vi "Find Controls Log Files for Shift.vi"(8 "error in (no error)":errorcluster, 10 "Date/Time":T1, 11 "Log File Directory":path=path "C:/Users/plane/Desktop/Data/runs-2014_11_21_16_00/runs") -> (0 "error out":errorcluster, 3 "Relevant Log Files":path[](array[path]))   [LabVIEW 2013, in "Controls Log Monitor.lvlib"]
uses:
  <vilib>/Utility/miscctls.llb/LVDateTimeRec.ctl
  Controls Log Monitor.lvlib
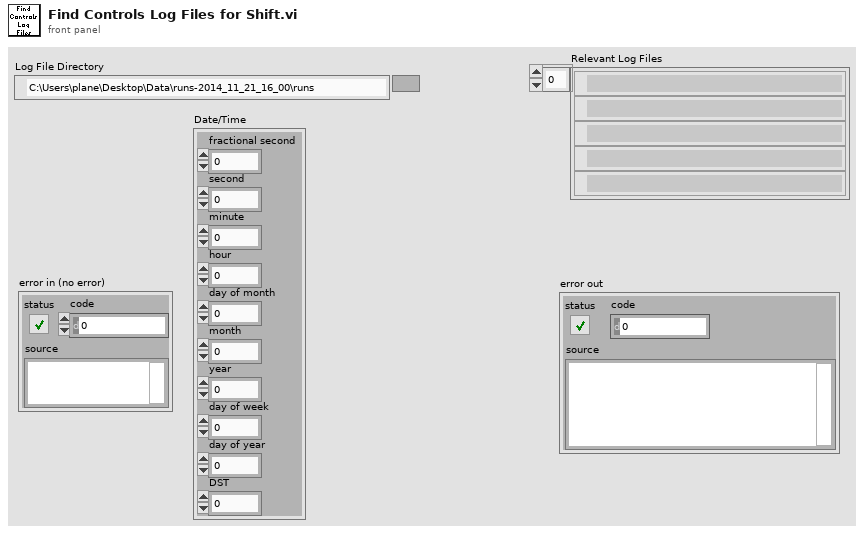
[diagram p1: front panel]
types:
  T1 = typedef "LVDateTimeRec.ctl" = cluster{"fractional second":dbl, "second":i32, "minute":i32, "hour":i32, "day of month":i32, "month":i32, "year":i32, "day of week":i32, "day of year":i32, "DST":i32}
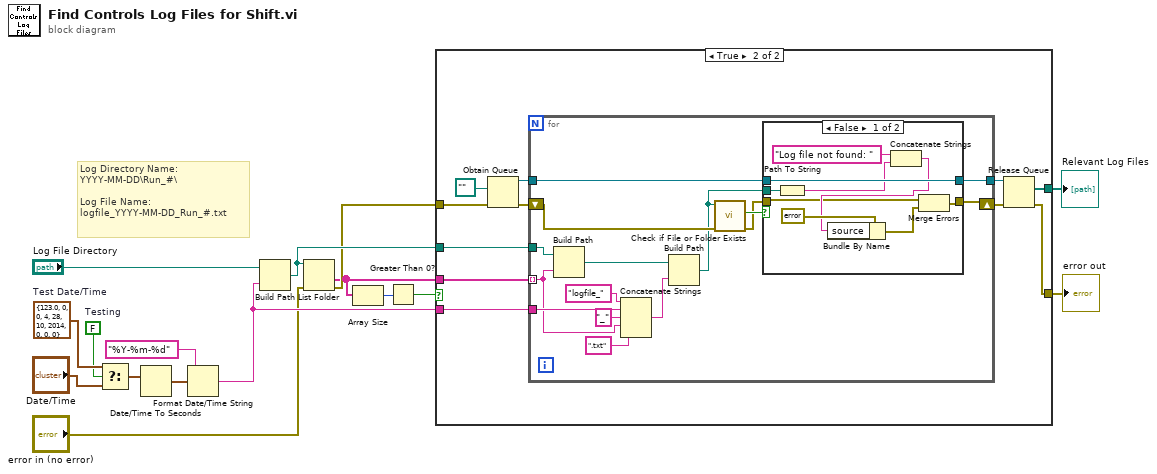
[diagram p0: block diagram]
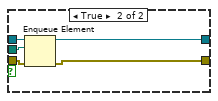
[diagram p3: hidden frame]
diagram:
  w7 = FALSE  # Testing
  w8 = T1 {"fractional second"=123.0, "second"=0, "minute"=0, "hour"=4, "day of month"=28, "month"=10, "year"=2014, "day of week"=0, "day of year"=0, "DST"=0}  # Test Date/Time
  # "Log Directory Name:\nYYYY-MM-DD\\Run_#\\\n\nLog File Name:\nlogfile_YYYY-MM-DD_Run_#.txt"
  n1 = Select(t=w8, s=w7, f="Date/Time") -> (s? t:f=w10:T1)
  n2 = Date/Time To Seconds(2:w10) -> (0:w16:timestamp)  [unwired: 1 in]
  n3 = Format Date/Time String(time format string (%c)="%Y-%m-%d", seconds (now)=w16) -> (date/time string=w12:string)  [unwired: 1 in]
  n4 = Build Path(base path="Log File Directory", name or relative path=w12) -> (appended path=w13:path)
  n5 = List Folder(path=w13, error in="error in (no error)") -> (folder names=w3:string[], error out=w5:errorcluster)  [unwired: 2 in, 2 out]
  n6 = Array Size(array=w3) -> (size(s)=w2:i32)
  n7 = Greater Than 0?(x=w2) -> (x > 0?=w1:bool)
  n8 = case shown="True" w1 {
    tunnel: w13 -> [_ w28]
    tunnel: w12 -> [_ w27]
    tunnel: [_ w21] -> w6
    tunnel: w5 -> [w17 w20]
    tunnel: [w17 w19] -> w4
    tunnel: w3 -> [_ w18]
    frame False {
    }
    frame True {
      n9 = Obtain Queue(element data type=path "" ("appended path"), error in (no error)=w20) -> (queue out=w25:refnum<queue>, error out=w24:errorcluster)  [unwired: 3 in, 1 out]
      n10 = for {
        tunnel: w18 -> [w39] mode=indexing
        tunnel: w28 -> [w43]
        tunnel: w27 -> [w41]
        tunnel: w25 -> [w35]
        tunnel: [w30] -> w23
        shift-right: [w29] -> w22
        shift-left: w24 -> [w34]
        n11 = Build Path(base path=w43, name or relative path=w39) -> (appended path=w37:path)
        n12 = Concatenate Strings("logfile_" ("string"), w41, "_" ("string"), w39, ".txt" ("string")) -> (w36:string)
        n13 = Build Path(base path=w37, name or relative path=w36) -> (appended path=w32:path)
        n14 = call <vilib>:"Check if File or Folder Exists.vi"("error in (no error)"=w34, "path"=w32) -> ("error out"=w31:errorcluster, "file or folder exists?"=w33:bool)  [unwired: 7 in, 1 out]
        n15 = case shown="False" w33 {
          tunnel: w35 -> [w52 w57]
          tunnel: w32 -> [w51 w56]
          tunnel: w31 -> [w45 w55]
          tunnel: [w52 w54] -> w30
          tunnel: [w46 w53] -> w29
          frame False {
            n16 = Path To String(path=w51) -> (string=w49:string)
            n17 = Concatenate Strings("Log file not found: " ("string"), w49) -> (w47:string)
            n18 = Bundle By Name(cluster=errorcluster {"status"=TRUE, "code"=7, "source"=""} ("error constant"), "source"=w47) -> (w44:errorcluster)
            n19 = Merge Errors(w45, w44) -> (w46:errorcluster)
          }
          frame True {
            n20 = Enqueue Element(queue=w57, element=w56, error in (no error)=w55) -> (queue out=w54:refnum<queue>, error out=w53:errorcluster)  [unwired: 1 in, 1 out]
          }
        }
      }
      n21 = Release Queue(queue=w23, error in (no error)=w22) -> (remaining elements=w21:path[], error out=w19:errorcluster)  [unwired: 1 in, 1 out]
    }
  }
  "Relevant Log Files" <- w6
  "error out" <- w4
